vi "GetMetadataValue.vi"(8 "error in (no error)":errorcluster, 10 "key":string, 11 "session id in":i32) -> (0 "error out":errorcluster, 1 "MetadataKey":string, 2 "GetMetadataKey":bool, 3 "session id out":i32)   [LabVIEW 2017, in "libonnx_wrapper.lvlib"]
doc: "/**\n * @brief Получить значение метаданных по ключу\n * \n * @param sessionId [IN] ID сессии\n * @param key [IN] Ключ метаданных (например, \"producer_name\")\n * @param buffer [OUT] Буфер для строки со значением\n * @param bufferSize [IN] Размер буфера (рекомендуется 256)\n * \n * @return int32: 0 при успехе\n * @return int32: -1 если ключ не найден\n */\nint GetMetadataValue(int sessionId, const char* key, char* buffer, int bufferSize);"
uses:
  libonnx_wrapper.lvlib
panel:
  out "bufferSize":i32
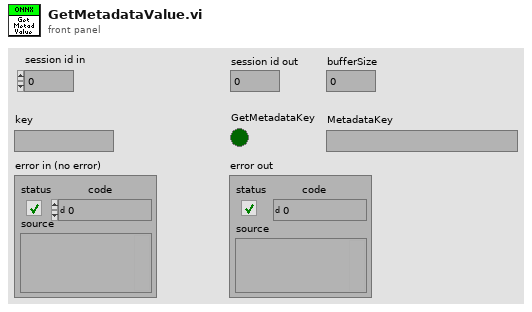
[diagram p1: front panel]
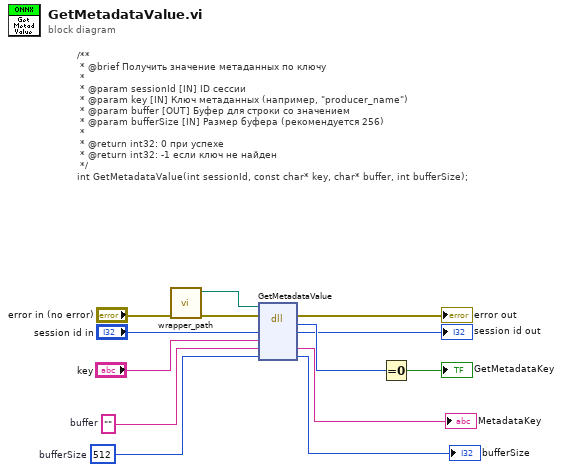
[diagram p0: block diagram]
diagram:
  w4 = 512  # bufferSize
  w5 = ""  # buffer
  # "/**\n * @brief Получить значение метаданных по ключу\n * \n * @param sessionId [IN] ID сессии\n * @param key [IN] Ключ метаданных (например, \"producer_name\")\n * @param buffer [OUT] Буфер для строки со значением\n * @param bufferSize [IN] Размер буфера (рекомендуется 256)\n * \n * @return int32: 0 при успехе\n * @return int32: -1 если ключ не найден\n */\nint GetMetadataValue(int sessionId, const char* key, char* buffer, int bufferSize);"
  n1 = call "wrapper_path.vi"("error in (no error)"="error in (no error)") -> ("error out"=w11:errorcluster, "wrapper path"=w10:path)  [unwired: 9 in]
  n2 = dll-call lib="home/ivan/LabVIEWData/ONNX/Test/libonnx_wrapper/unix64/libonnx_wrapper.*" fn="GetMetadataValue"(path in=w10, error in=w11, "sessionId"="session id in", "key"="key", "buffer"=w5, "bufferSize"=w4) -> (error out=→"error out":errorcluster, "GetMetadataValue"=w7:i32, "sessionId"=→"session id out":i32, "buffer"=→"MetadataKey":string, "bufferSize"=→"bufferSize":i32)  [unwired: 2 in, 1 out]
  n3 = Equal To 0?(x=w7) -> (x = 0?=→"GetMetadataKey":bool)
